vi "GDSIconEditor_HeaderEditorDialog.vi"(1 "BodyBackGround":u32(colorbox), 2 "HeaderText":string, 5 "error in (no error)":errorcluster, 6 "HeaderIconIn":u8[][](array[numeric]) format="%x", 7 "Type":T2, 8 "FrameThickness(1)":u32=1, 9 "ClassBodyIcon":string, 10 "FrameColor":u32(colorbox)) -> (15 "Cancelled":bool, 16 "FrameColorOut":u32(colorbox), 17 "FrameThicknessOut":u32=1, 18 "HeaderIconOut":u8[][](array[numeric]) format="%x", 19 "error out":errorcluster)   [LabVIEW 2020]
uses:
  <resource>/Framework/Providers/Open_GDS/ClassProviders/Common/LvIcon_class/GDSLvIcon_ColorControl.ctl
  <resource>/Framework/Providers/Open_GDS/ClassProviders/Common/LvIcon_class/GDSLvIcon_Type.ctl
  <vilib>/Utility/miscctls.llb/LVPoint32TypeDef.ctl
  <resource>/Framework/Providers/Open_GDS/ClassProviders/Common/LvIcon_class/GDSLvIcon_ClassColorTypes.ctl
  <resource>/Framework/Providers/Open_GDS/ClassProviders/Common/LvIcon_class/subvis/GDSLvIcon_TextDataType.ctl
  <resource>/Framework/Providers/Open_GDS/ClassProviders/Common/LvIcon_class/GDSLvIcon_WordCompressionType.ctl
  <resource>/Framework/Providers/Open_GDS/ClassProviders/Common/LvIcon_class/GDSLvIcon_TextAlignment.ctl
  <vilib>/event_ctls.llb/lveventtype.ctl
  <vilib>/Analysis/NI_AALBase.lvlib
panel:
  out "Coords 2":T1
  out "Coords":T1
  in  "_LastHeaders":picture[](array[picture]) caption="Last used headers"
  in  "Help":bool
  in  "Dice":cluster{"Boolean 2":bool, "Dice 2":bool}
  out "Icon Preview":picture
  in  "Frame":T3 caption="Color"
  in  "Thickness (pixels)":u8=3 min=1 max=3 step=1
  in  "Rows":enum16{"1 Row", "2 Rows", "3 Rows"}(ring)
  in  "Font Compression":enum16{"Auto", "On", "Off"}(ring)
  in  "CapitalOnly":bool=TRUE caption="Only use capital characters"
  in  "Height (pixels)":u8=9 min=5 max=19
  in  "Text":string="Endevo"
  in  "HeaderBk":T3 caption="Background"
  in  "HeaderText":T3 caption="Text"
  in  "OK":bool
  in  "Cancel":bool
  # "Header"
  # "Random color generation"
  # "Frame"
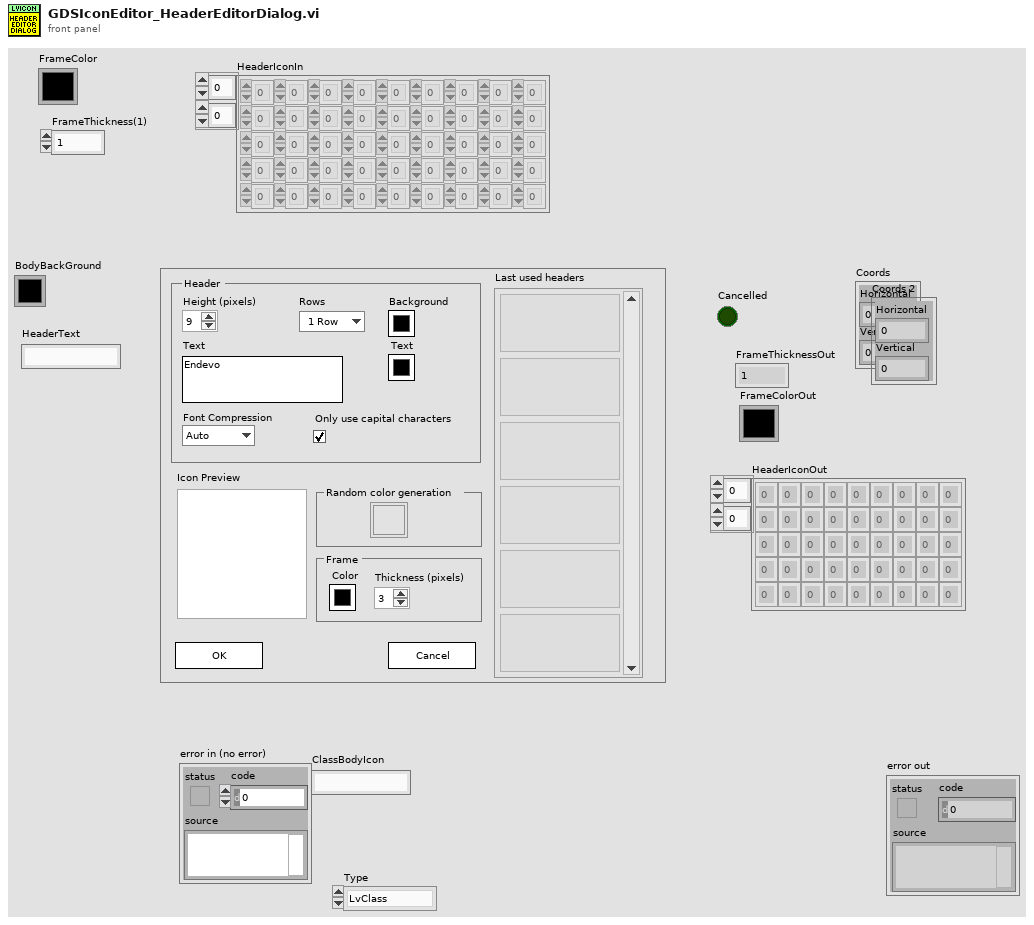
[diagram p1: front panel]
types:
  T1 = typedef "LVPoint32TypeDef.ctl" = cluster{"Horizontal":i32, "Vertical":i32}
  T2 = typedef "GDSLvIcon_Type.ctl" = enum16{"LvClass", "Library", "X-Control", "LvInterface"}
  T3 = typedef "GDSLvIcon_ColorControl.ctl" = cluster{"Decal":bool, "Color":u32}
  T4 = cluster{"Names":string[], "Headers":cluster{"Header":u8[][]}[]}
  T5 = typedef "GDSLvIcon_ClassColorTypes.ctl" = cluster{"Frame":u32, "Header Text Color":u32, "Header Background":u32, "BodyBackgroundPublic":u32, "BodyBackgroundProtected":u32, "BodyBackgroundPrivate":u32, "Body Text Color":u32, "Frame thickness":u8, "ProtectedPrivateSame":bool, "Icon Header Size":u8, "Font Compression":enum16{"Auto", "On", "Off"}, "CapitalOnly":bool}
  T6 = cluster{"Header":u8[][], "Cancel":bool, "Names":string[], "Headers":cluster{"Header":u8[][]}[]}
  T7 = cluster{"Selection Start":u32, "Selection End":u32}
  T8 = cluster{"left":i16, "top":i16, "right":i16, "bottom":i16}
  T9 = typedef "GDSLvIcon_TextDataType.ctl" = cluster{"Text":string, "Allow Only Capital Chars":bool, "Compression":T10, "Alignment":T11}
  T10 = typedef "GDSLvIcon_WordCompressionType.ctl" = enum16{"Auto", "On", "Off"}
  T11 = typedef "GDSLvIcon_TextAlignment.ctl" = enum16{"Center", "Left", "Right"}
  T12 = typedef "lveventtype.ctl" = enum32{"Null", "Timeout", "Annotation Menu Selection", "Annotation Menu Selection?", "App Instance Close", "App Instance Close?", "Autoscale Range Change", "Bookmark Info Change", "Cell Edit", "Cell Edit?", "Cursor Grab", "Cursor Grab?", "Cursor Menu Selection", "Cursor Menu Selection?", "Cursor Move", "Cursor Release", "Data Change", "Direction Change", "Display State Change", "Drag Ended", "Drag Enter", "Drag Leave", "Drag Over", "Drag Source Update", "Drag Starting", "Drag Starting?", "Drop", "Exec State Change", "Key Down", "Key Down?", "Key Repeat", "Key Repeat?", "Key Up", "Listbox Double Click", "Menu Activation?", "Menu Selection (App)", "Menu Selection? (App)", "Menu Selection (User)", "Mouse Down", "Mouse Down?", "Mouse Enter", "Mouse Leave", "Mouse Move", "Mouse Up", "Mouse Wheel", "NI Security User Change (App)", "Pane Size", "Panel Close", "Panel Close?", "Panel Resize", "Plot Attribute Change", "Scale Range Change", "Shortcut Menu Activation?", "Shortcut Menu Selection (App)", "Shortcut Menu Selection? (App)", "Shortcut Menu Selection (User)", "Tree Double Click", "Tree Drag", "Tree Drag?", "Tree Drop", "Tree Drop?", "Tree Item Close", "Tree Item Close?", "Tree Item Open", "Tree Item Open?", "User Event", "Value Change"}
  T13 = typedef "ColorControl.ctl" = cluster{"Decal":bool, "Color":u32}
  T14 = typedef "LVRectTypeDef.ctl" = cluster{"Left":i16, "Top":i16, "Right":i16, "Bottom":i16}
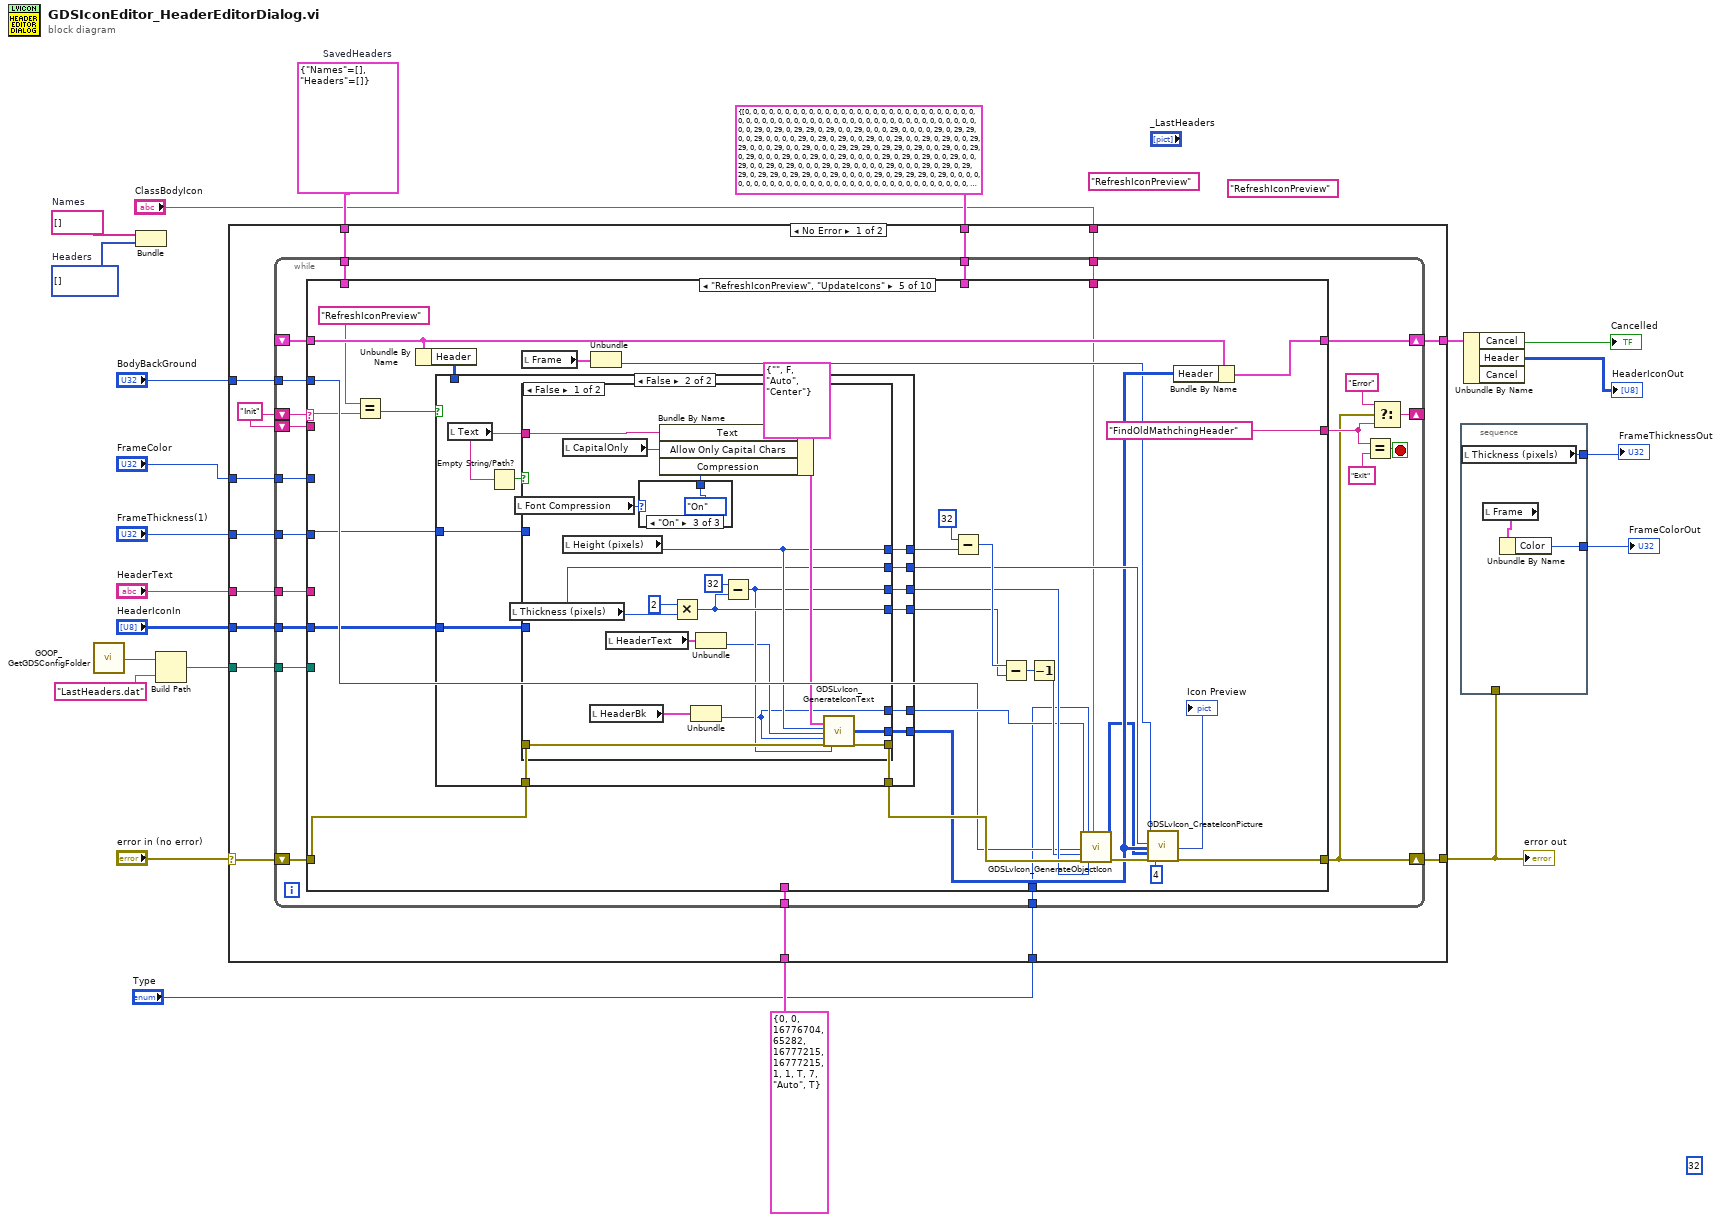
[diagram p0: block diagram]
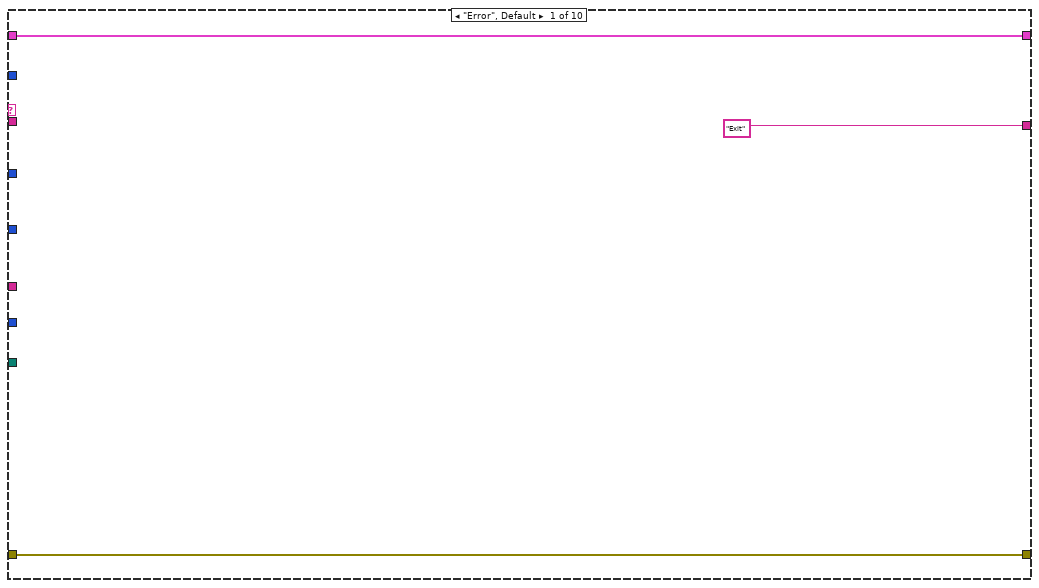
[diagram p2: hidden frame]
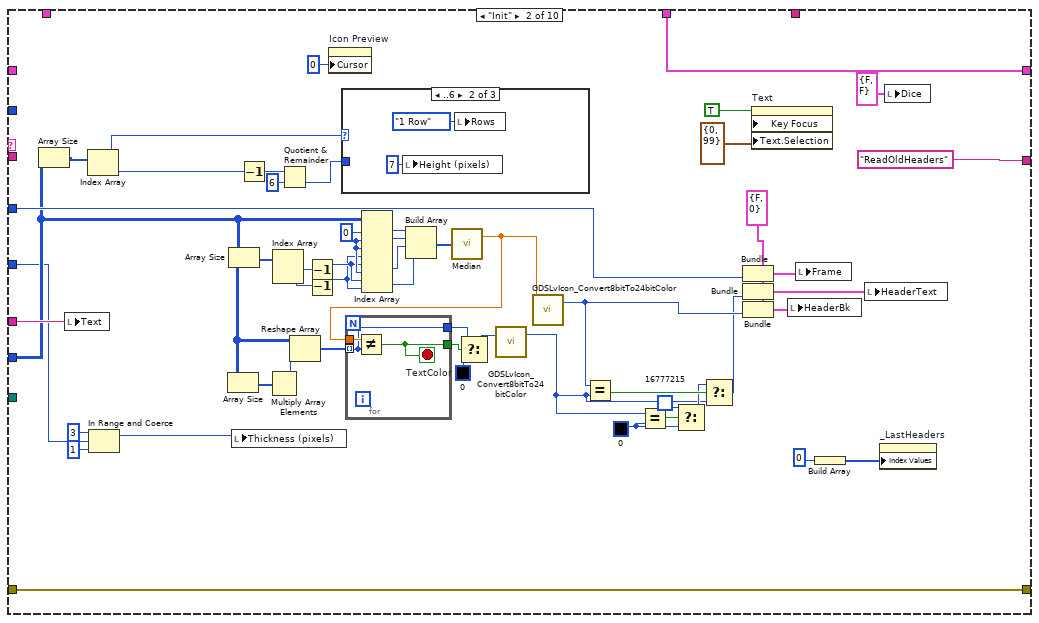
[diagram p3: hidden frame]
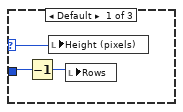
[diagram p4: hidden frame]
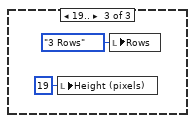
[diagram p5: hidden frame]
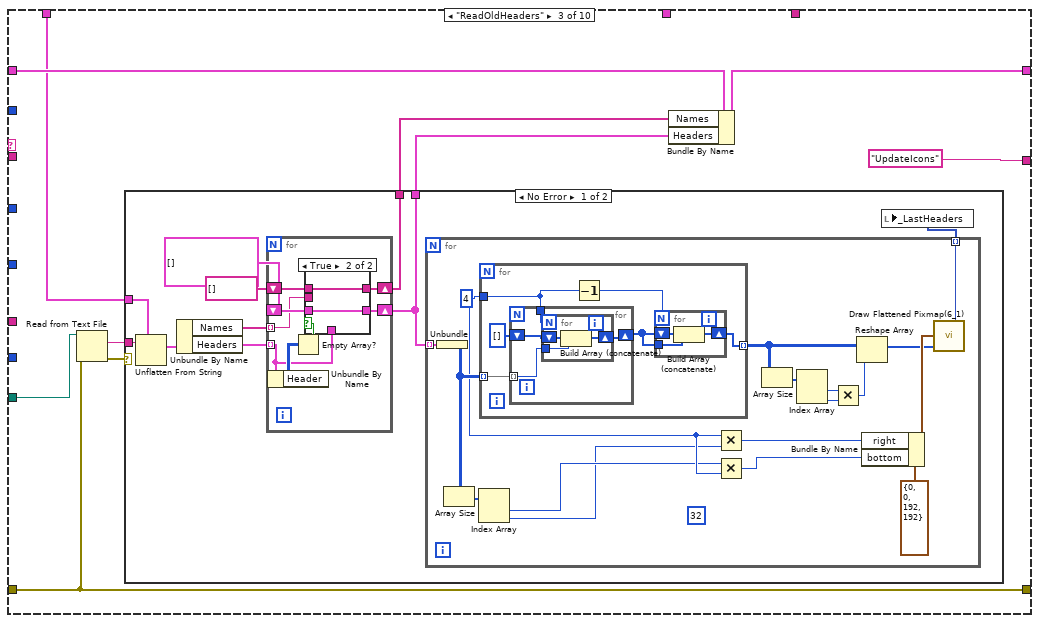
[diagram p6: hidden frame]
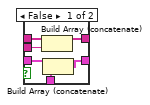
[diagram p7: hidden frame]
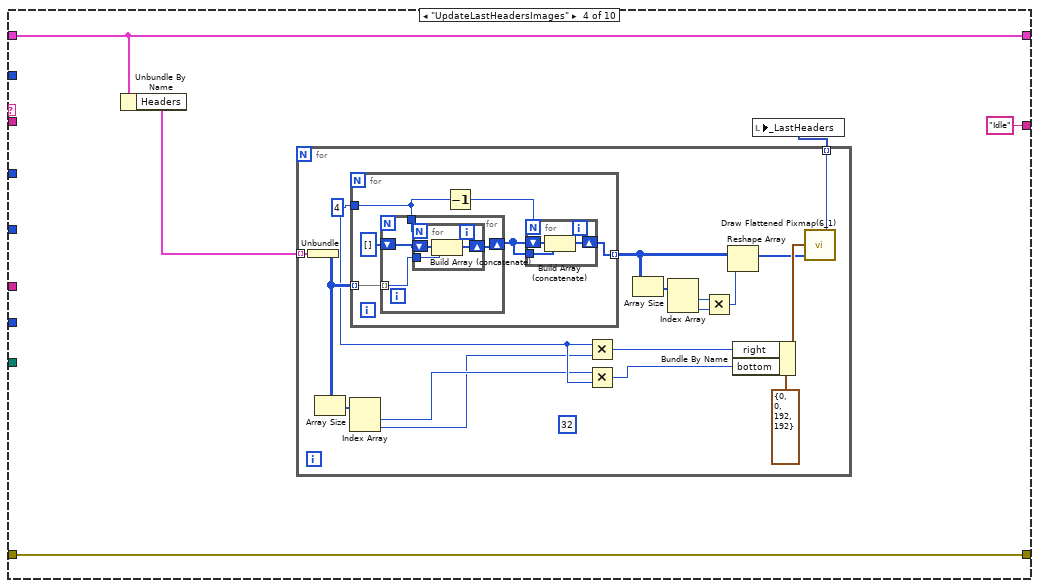
[diagram p9: hidden frame]
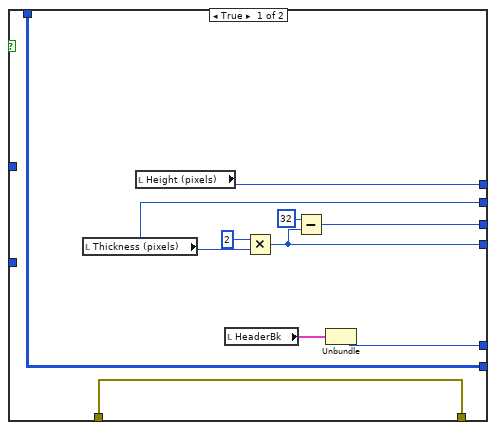
[diagram p10: hidden frame]
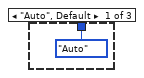
[diagram p11: hidden frame]
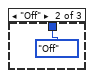
[diagram p12: hidden frame]
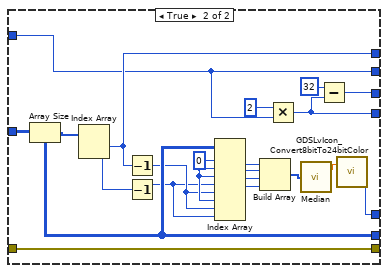
[diagram p13: hidden frame]
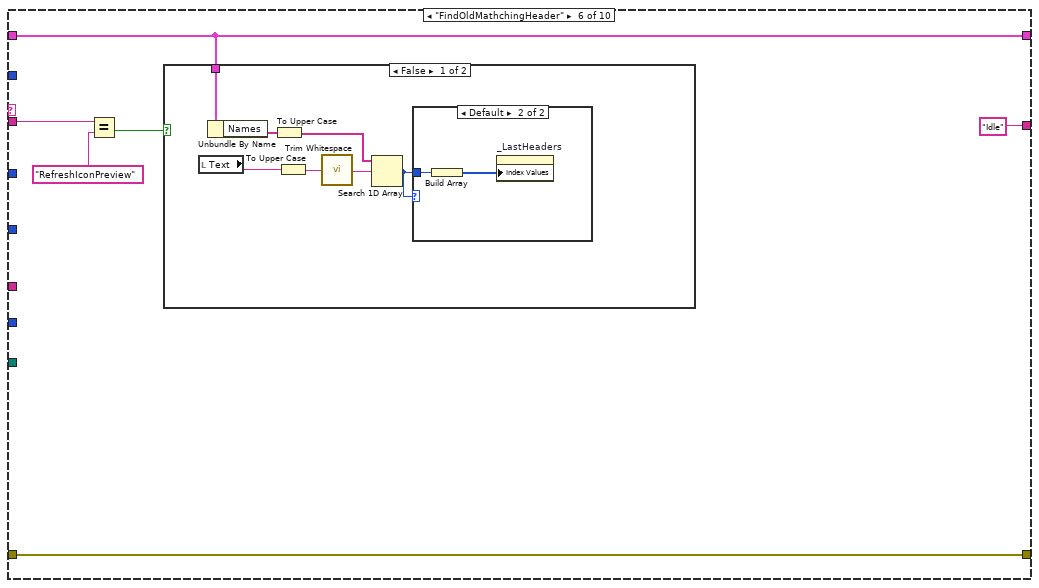
[diagram p14: hidden frame]
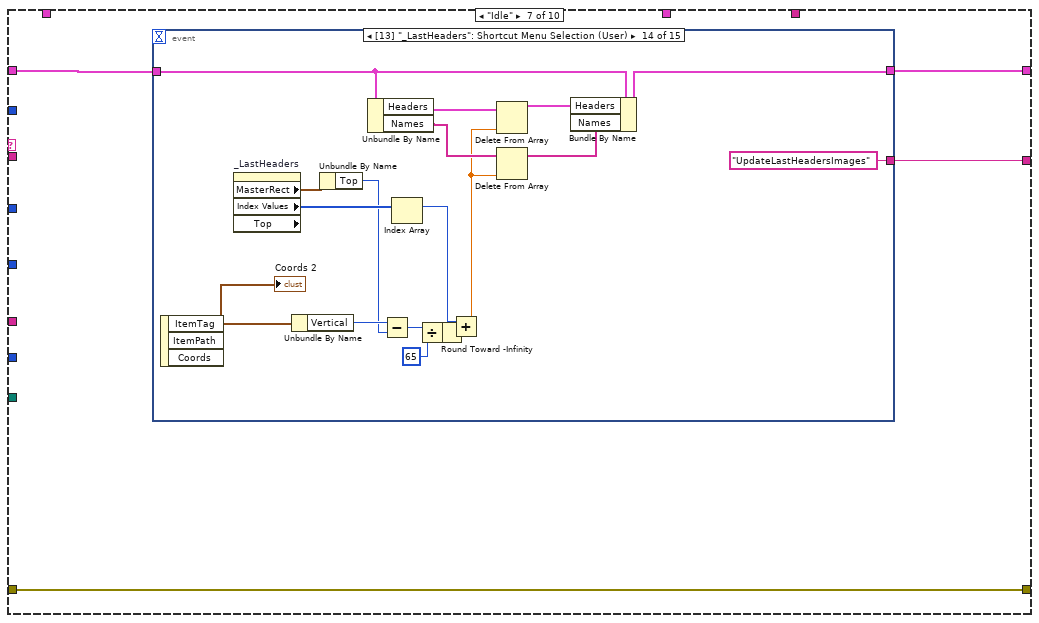
[diagram p17: hidden frame]
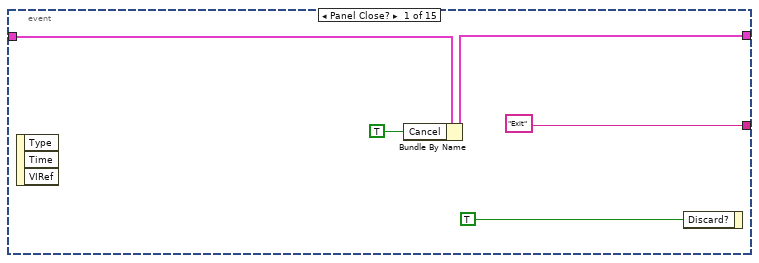
[diagram p18: hidden frame]
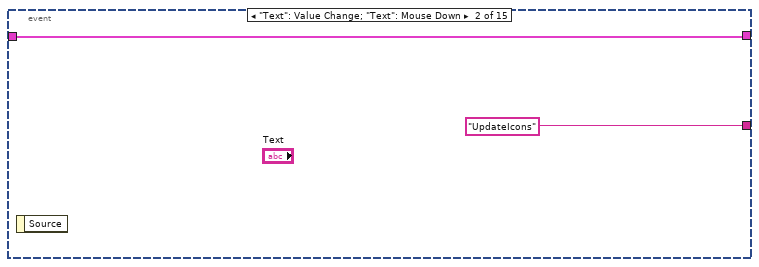
[diagram p19: hidden frame]
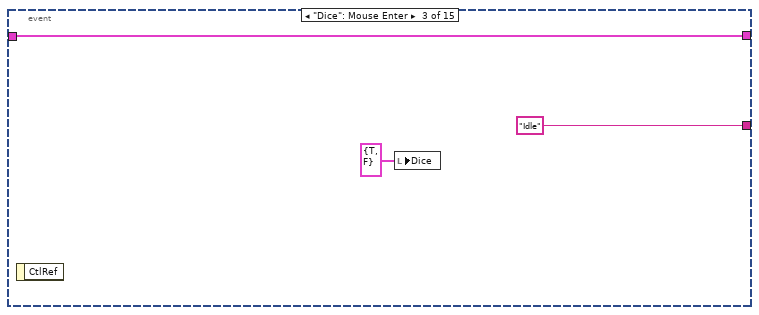
[diagram p20: hidden frame]
diagram:
  (unwired) "RefreshIconPreview"
  (unwired) "RefreshIconPreview"
  w2 = T4 {"Names"=[], "Headers"=[]}  # SavedHeaders
  (unwired) i16 32 ("bottom")
  w4 = picture[] []  # Headers
  w3 = string[] []  # Names
  n1 = call <resource>:"GOOP_GetGDSConfigFolder.vi"() -> ("GDSFolderPath"=w6:path)
  n2 = Bundle("Names"=w3, "Headers"=w4) -> ()  [unwired: 1 in, 1 out]
  n3 = Build Path(base path=w6, name or relative path="LastHeaders.dat") -> (appended path=w5:path)
  n4 = case shown="No Error" "error in (no error)" {
    selector: "error in (no error)" -> [w37 w575]
    tunnel: [w36 w575] -> w12
    tunnel: "BodyBackGround" -> [w35 _]
    tunnel: T6 {"Header"=[[0, 0, 0, 0, 0, 0, 0, 0, 0, 0, 0, 0, 0, 0, 0, 0, 0, 0, 0, 0, 0, 0, 0, 0, 0, 0, 0, 0, 0, 0], [0, 0, 0, 0, 0, 0, 0, 0, 0, 0, 0, 0, 0, 0, 0, 0, 0, 0, 0, 0, 0, 0, 0, 0, 0, 0, 0, 0, 0, 0], [0, 29, 0, 29, 0, 29, 29, 0, 29, 0, 0, 29, 0, 0, 0, 29, 0, 0, 0, 0, 29, 0, 29, 29, 0, 0, 29, 0, 0, 0], [0, 29, 0, 29, 0, 29, 0, 0, 29, 0, 0, 29, 0, 0, 29, 0, 29, 0, 0, 29, 29, 0, 0, 0, 29, 0, 0, 29, 0, 0], [0, 29, 29, 29, 0, 29, 29, 0, 29, 0, 0, 29, 0, 0, 29, 0, 29, 0, 0, 0, 29, 0, 0, 29, 0, 0, 29, 0, 0, 0], [0, 29, 0, 29, 0, 29, 0, 0, 29, 0, 0, 29, 0, 0, 29, 0, 29, 0, 0, 0, 29, 0, 29, 0, 0, 0, 0, 29, 0, 0], [0, 29, 0, 29, 0, 29, 29, 0, 29, 29, 0, 29, 29, 0, 0, 29, 0, 0, 0, 0, 29, 0, 29, 29, 29, 0, 29, 0, 0, 0], [0, 0, 0, 0, 0, 0, 0, 0, 0, 0, 0, 0, 0, 0, 0, 0, 0, 0, 0, 0, 0, 0, 0, 0, 0, 0, 0, 0, 0, 0], [0, 0, 0, 0, 0, 0, 0, 0, 0, 0, 0, 0, 0, 0, 0, 0, 0, 0, 0, 0, 0, 0, 0, 0, 0, 0, 0, 0, 0, 0]], "Cancel"=FALSE, "Names"=[], "Headers"=[]} -> [w34 _]
    tunnel: T5 {"Frame"=0, "Header Text Color"=0, "Header Background"=16776704, "BodyBackgroundPublic"=65282, "BodyBackgroundProtected"=16777215, "BodyBackgroundPrivate"=16777215, "Body Text Color"=1, "Frame thickness"=1, "ProtectedPrivateSame"=TRUE, "Icon Header Size"=7, "Font Compression"=enum."Auto", "CapitalOnly"=TRUE} ("type") -> [w33 _]
    tunnel: "FrameThickness(1)" -> [w32 _]
    tunnel: "FrameColor" -> [w31 _]
    tunnel: "HeaderText" -> [w30 _]
    tunnel: [w29 _] -> w15
    tunnel: "HeaderIconIn" -> [w28 _]
    tunnel: "Type" -> [w27 _]
    tunnel: w5 -> [w26 _]
    tunnel: w2 -> [w25 _]
    tunnel: "ClassBodyIcon" -> [w23 _]
    frame No Error {
      w24 = "Init"
      n5 = while {
        shift-right: [w52] -> w36
        shift-left: w37 -> [w59]
        shift-right: [w57] -> _
        shift-left: w24 -> [w58]
        shift-right: [w41] -> w29
        shift-left: _ -> [w51]
        tunnel: w35 -> [w50]
        tunnel: w34 -> [w49]
        tunnel: w33 -> [w48]
        tunnel: w32 -> [w47]
        tunnel: w31 -> [w46]
        tunnel: w30 -> [w45]
        tunnel: w28 -> [w44]
        tunnel: w27 -> [w43]
        tunnel: w26 -> [w42]
        tunnel: w25 -> [w40]
        shift-left: w24 -> [w39]
        tunnel: w23 -> [w38]
        stop <- w56 stop-if-true
        n6 = case shown="\"RefreshIconPreview\", \"UpdateIcons\"" w58 {
          selector: w58 -> [_ _ _ _ w236 _ _ _ _ _]
          tunnel: w59 -> [w62 w105 w127 w197 w262 w330 w344 w457 w515 w532]
          tunnel: [w62 w105 w127 w197 w254 w330 w344 w457 w515 w532] -> w52
          tunnel: ["Exit" "ReadOldHeaders" "UpdateIcons" "Idle" "FindOldMathchingHeader" "Idle" w345 "RefreshIconPreview" "UpdateIcons" "Exit"] -> w53
          tunnel: w51 -> [w60 _ w130 w195 w237 w331 w343 w489 w530 w540]
          tunnel: w50 -> [_ _ _ _ w241 _ _ _ _ _]
          tunnel: w49 -> [_ w104 _ _ _ _ _ _ _ _]
          tunnel: w48 -> [_ _ _ _ _ _ _ _ _ _]
          tunnel: w47 -> [_ w69 _ _ w239 _ _ _ _ _]
          tunnel: w46 -> [_ w108 _ _ _ _ _ _ _ _]
          tunnel: w45 -> [_ w103 _ _ _ _ _ _ _ _]
          tunnel: w44 -> [_ w75 _ _ w240 _ _ _ _ _]
          tunnel: w43 -> [_ _ _ _ w238 _ _ _ _ _]
          tunnel: w42 -> [_ _ w133 _ _ _ _ _ _ w534]
          tunnel: [w60 w104 w129 w195 w248 w331 w342 w489 w530 w540] -> w41
          tunnel: w40 -> [_ _ w125 _ _ _ _ _ _ w535]
          tunnel: w39 -> [_ _ _ _ _ w329 _ _ _ _]
          tunnel: w38 -> [_ _ _ _ w233 _ _ _ _ _]
          frame "Error", Default {
          }
          frame "Init" {
            w109 = T3 {"Decal"=FALSE, "Color"=0} ("Frame")
            w76 = u32 0  # TextColor
            w90 = 0 ("index (row)")
            w70 = u32 0
            n7 = Array Size(array=w75) -> (size(s)=w102:i32[])
            n8 = local write "Text"(w103) -> ()
            n9 = Index Array(array=w102) -> (element=w99:i32)  [unwired: 1 in]
            n10 = In Range and Coerce(upper limit=u32 3, x=w69, lower limit=u32 1) -> (coerced(x)=w66:u32)  [unwired: 1 out]
            n11 = Array Size(array=w75) -> (size(s)=w82:i32[])
            n12 = Array Size(array=w75) -> (size(s)=w93:i32[])
            n13 = local write "Thickness (pixels)"(w66) -> ()
            n14 = Decrement(x=w99) -> (x-1=w101:i32)
            n15 = Multiply Array Elements(1:w82) -> (0:w80:i32)
            n16 = Index Array(array=w93) -> (element #1=w92:i32, element #2=w91:i32)  [unwired: 2 in]
            n17 = Quotient & Remainder(x=w101, y=6) -> (floor(x/y)=w98:i32)  [unwired: 1 out]
            n18 = Reshape Array(w75, w80) -> (w81:u8[])
            n19 = Decrement(x=w92) -> (x-1=w89:i32)
            n20 = Decrement(x=w91) -> (x-1=w88:i32)
            n21 = property on="Icon Preview" class="Pict"("Cursor"=0) -> ()  [unwired: 2 in, 2 out]
            n22 = case shown="..6" w99 {
              selector: w99 -> [w120 _ _]
              tunnel: w98 -> [w119 _ _]
              frame Default {
                n23 = Decrement(x=w119) -> (x-1=w118:i32)
                n24 = local write "Height (pixels)"(w120) -> ()
                n25 = local write "Rows"(w118) -> ()
              }
              frame ..6 {
                n26 = local write "Height (pixels)"(u8 7 ("Height (pixels)")) -> ()
                n27 = local write "Rows"(enum16{"1 Row", "2 Rows", "3 Rows"}."1 Row" ("Rows")) -> ()
              }
              frame 19.. {
                n28 = local write "Height (pixels)"(u8 19 ("Height (pixels)")) -> ()
                n29 = local write "Rows"(enum16{"1 Row", "2 Rows", "3 Rows"}."3 Rows" ("Rows")) -> ()
              }
            }
            n30 = Index Array(array=w75, index (row) #1=w90, index (col) #1=w90, index (row) #2=w90, index (col) #2=w88, index (row) #3=w89, index (col) #3=w90, index (row) #4=w89, index (col) #4=w88) -> (element #1=w87:u8, element #2=w86:u8, element #3=w85:u8, element #4=w84:u8)
            n31 = Build Array(w87, w86, w85, w84) -> (w83:u8[])
            n32 = call <vilib>:"Median.vi"("X"=w83) -> ("median"=w74:dbl)  [unwired: 1 out]
            n33 = for {
              tunnel: w81 -> [w116] mode=indexing
              tunnel: w74 -> [w117]
              tunnel: [w115] -> w78
              tunnel: [w116] -> w77
              stop <- w115 stop-if-true
              n34 = Not Equal?(x=w117, y=w116) -> (x != y?=w115:bool)
            }
            n35 = Select(t=w77, s=w78, f=w76) -> (s? t:f=w79:u32)
            n36 = call <resource>:"GDSLvIcon_Convert8bitTo24bitColor.vi"("Color8bit"=w79) -> ("Color24bit"=w71:u32)  [unwired: 17 in, 1 out]
            n37 = call <resource>:"GDSLvIcon_Convert8bitTo24bitColor.vi"("Color8bit"=w74) -> ("Color24bit"=w73:u32)  [unwired: 17 in, 1 out]
            n38 = Equal?(x=w73, y=w71) -> (x = y?=w97:bool)
            n39 = Equal?(x=w71, y=w70) -> (x = y?=w96:bool)
            n40 = Select(t=u32 16777215, s=w96, f=w70) -> (s? t:f=w94:u32)
            n41 = Select(t=w94, s=w97, f=w71) -> (s? t:f=w72:u32)
            n42 = Bundle(cluster=w109, "Color"=w108) -> (w112:T3)  [unwired: 1 in]
            n43 = Bundle(cluster=w109, "Color"=w72) -> (w111:T3)  [unwired: 1 in]
            n44 = Bundle(cluster=w109, "Color"=w73) -> (w110:T3)  [unwired: 1 in]
            n45 = property on="Text" class="Str"("Key Focus"=TRUE, "Text.Selection"=T7 {"Selection Start"=0, "Selection End"=99}) -> ()  [unwired: 2 in, 2 out]
            n46 = local write "HeaderBk"(w110) -> ()
            n47 = local write "Frame"(w112) -> ()
            n48 = Build Array(u32 0) -> (w65:u32[])
            n49 = local write "HeaderText"(w111) -> ()
            n50 = property on="_LastHeaders" class="Arr (strict)"("Index Values"=w65) -> ()  [unwired: 2 in, 2 out]
            n51 = local write "Dice"(cluster{"Boolean 2":bool, "Dice":bool} {"Boolean 2"=FALSE, "Dice"=FALSE} ("Dice")) -> ()
          }
          frame "ReadOldHeaders" {
            n52 = Read from Text File(file (use dialog)=w133, error in=w127) -> (text=w131:string, error out=w132:errorcluster)  [unwired: 2 in, 2 out]
            n53 = case shown="No Error" w132 {
              tunnel: w131 -> [w144 _]
              tunnel: w125 -> [w143 _]
              tunnel: [w135 _] -> w128
              tunnel: [w136 _] -> w126
              frame No Error {
                n54 = Unflatten From String(type=w143, binary string=w144) -> (value=w142:T4)  [unwired: 3 in, 2 out]
                n55 = Unbundle By Name(w142) -> ("Names"=w140:string[], "Headers"=w139:cluster{"Header":u8[][]}[])
                n56 = for {
                  tunnel: w140 -> [w147] mode=indexing
                  tunnel: w139 -> [w145] mode=indexing
                  shift-right: [w148] -> w135
                  shift-left: string[] [] -> [w150]
                  shift-right: [w146] -> w136
                  shift-left: cluster{"Header":u8[][]}[] [] -> [w149]
                  n57 = Unbundle By Name(w145) -> ("Header"=w152:u8[][])
                  n58 = Empty Array?(array=w152) -> (empty?=w151:bool)
                  n59 = case shown="True" w151 {
                    tunnel: w150 -> [w157 w159]
                    tunnel: w149 -> [w155 w160]
                    tunnel: [w158 w159] -> w148
                    tunnel: w147 -> [w156 _]
                    tunnel: [w154 w160] -> w146
                    tunnel: w145 -> [w153 _]
                    frame False {
                      n60 = Build Array (concatenate)(w157, w156) -> (w158:string[])
                      n61 = Build Array (concatenate)(w155, w153) -> (w154:cluster{"Header":u8[][]}[])
                    }
                    frame True {
                    }
                  }
                }
                n62 = for {
                  tunnel: w136 -> [w177] mode=indexing
                  tunnel: [w167] -> w141 mode=indexing
                  w164 = 4 ("BigSizeIcon(x6)")
                  (unwired) 32 ("y")
                  n63 = Unbundle(w177) -> ("Header"=w165:u8[][])
                  n64 = Array Size(array=w165) -> (size(s)=w166:i32[])
                  n65 = Index Array(array=w166) -> (element #1=w162:i32, element #2=w161:i32)  [unwired: 2 in]
                  n66 = for {
                    tunnel: w165 -> [w183] mode=indexing
                    tunnel: [w181] -> w172 mode=indexing
                    tunnel: w164 -> [w178]
                    n67 = for {
                      tunnel: w183 -> [w190] mode=indexing
                      shift-right: [w188] -> w180
                      shift-left: u8[] [] -> [w189]
                      tunnel: w178 -> [w187]
                      n68 = for {
                        N: w187 -> [_]
                        tunnel: w190 -> [w193]
                        shift-right: [w191] -> w188
                        shift-left: w189 -> [w192]
                        n69 = Build Array (concatenate)(w192, w193) -> (w191:u8[])
                      }
                    }
                    n70 = Decrement(x=w178) -> (x-1=w179:i32)
                    n71 = for {
                      N: w179 -> [_]
                      tunnel: w180 -> [w186]
                      shift-right: [w184] -> w181
                      shift-left: w180 -> [w185]
                      n72 = Build Array (concatenate)(w185, w186) -> (w184:u8[])
                    }
                  }
                  n73 = Multiply(x=w164, y=w161) -> (x*y=w176:i32)
                  n74 = Multiply(x=w162, y=w164) -> (x*y=w163:i32)
                  n75 = Array Size(array=w172) -> (size(s)=w168:i32[])
                  n76 = Index Array(array=w168) -> (element #1=w170:i32, element #2=w169:i32)  [unwired: 2 in]
                  n77 = Multiply(x=w170, y=w169) -> (x*y=w171:i32)
                  n78 = Reshape Array(w172, w171) -> (w173:u8[])
                  n79 = Bundle By Name(cluster=T8 {"left"=0, "top"=0, "right"=192, "bottom"=192} ("rect"), "right"=w176, "bottom"=w163) -> (w175:T8)
                  n80 = call <vilib>:"Draw Flattened Pixmap(6_1).vi"("rect"=w175, "flattened pixmap data"=w173) -> ("new picture"=w167:picture)  [unwired: 7 in]
                }
                n81 = local write "_LastHeaders"(w141) -> ()
              }
              frame Error {
              }
            }
            n82 = Bundle By Name(cluster=w130, "Names"=w128, "Headers"=w126) -> (w129:T6)
          }
          frame "UpdateLastHeadersImages" {
            n83 = Unbundle By Name(w195) -> ("Headers"=w196:cluster{"Header":u8[][]}[])
            n84 = for {
              tunnel: w196 -> [w215] mode=indexing
              tunnel: [w205] -> w198 mode=indexing
              w202 = 4 ("BigSizeIcon(x6)")
              (unwired) 32 ("y")
              n85 = Unbundle(w215) -> ("Header"=w203:u8[][])
              n86 = Array Size(array=w203) -> (size(s)=w204:i32[])
              n87 = Index Array(array=w204) -> (element #1=w200:i32, element #2=w199:i32)  [unwired: 2 in]
              n88 = for {
                tunnel: w203 -> [w221] mode=indexing
                tunnel: [w219] -> w210 mode=indexing
                tunnel: w202 -> [w216]
                n89 = for {
                  tunnel: w221 -> [w228] mode=indexing
                  shift-right: [w226] -> w218
                  shift-left: u8[] [] -> [w227]
                  tunnel: w216 -> [w225]
                  n90 = for {
                    N: w225 -> [_]
                    tunnel: w228 -> [w231]
                    shift-right: [w229] -> w226
                    shift-left: w227 -> [w230]
                    n91 = Build Array (concatenate)(w230, w231) -> (w229:u8[])
                  }
                }
                n92 = Decrement(x=w216) -> (x-1=w217:i32)
                n93 = for {
                  N: w217 -> [_]
                  tunnel: w218 -> [w224]
                  shift-right: [w222] -> w219
                  shift-left: w218 -> [w223]
                  n94 = Build Array (concatenate)(w223, w224) -> (w222:u8[])
                }
              }
              n95 = Multiply(x=w202, y=w199) -> (x*y=w214:i32)
              n96 = Multiply(x=w200, y=w202) -> (x*y=w201:i32)
              n97 = Array Size(array=w210) -> (size(s)=w206:i32[])
              n98 = Index Array(array=w206) -> (element #1=w208:i32, element #2=w207:i32)  [unwired: 2 in]
              n99 = Multiply(x=w208, y=w207) -> (x*y=w209:i32)
              n100 = Reshape Array(w210, w209) -> (w211:u8[])
              n101 = Bundle By Name(cluster=T8 {"left"=0, "top"=0, "right"=192, "bottom"=192} ("rect"), "right"=w214, "bottom"=w201) -> (w213:T8)
              n102 = call <vilib>:"Draw Flattened Pixmap(6_1).vi"("rect"=w213, "flattened pixmap data"=w211) -> ("new picture"=w205:picture)  [unwired: 7 in]
            }
            n103 = local write "_LastHeaders"(w198) -> ()
          }
          frame "RefreshIconPreview", "UpdateIcons" {
            n104 = Equal?(x="RefreshIconPreview", y=w236) -> (x = y?=w232:bool)
            n105 = Unbundle By Name(w237) -> ("Header"=w234:u8[][])
            n106 = case shown="False" w232 {
              tunnel: w262 -> [w266 w284]
              tunnel: [w266 w283] -> w260
              tunnel: [w272 w282] -> w256
              tunnel: [w271 w281] -> w252
              tunnel: [w270 w280] -> w251
              tunnel: [w269 w279] -> w250
              tunnel: [w265 w278] -> w247
              tunnel: [w263 w277] -> w243
              tunnel: w240 -> [_ w274]
              tunnel: w239 -> [_ w273]
              tunnel: w234 -> [w265 _]
              frame True {
                n107 = local read "Thickness (pixels)"() -> (w270:u8)
                n108 = local read "Height (pixels)"() -> (w272:u8)
                n109 = local read "HeaderBk"() -> (w264:T3)
                n110 = Multiply(x=u8 2, y=w270) -> (x*y=w271:u8)
                n111 = Subtract(x=32, y=w271) -> (x-y=w269:i32)
                n112 = Unbundle(w264) -> ("Color"=w263:u32)  [unwired: 1 out]
              }
              frame False {
                n113 = local read "Text"() -> (w275:string)
                n114 = Empty String/Path?(string/path=w275) -> (empty?=w276:bool)
                n115 = case shown="False" w276 {
                  tunnel: w284 -> [w303 w326]
                  tunnel: [w298 w326] -> w283
                  tunnel: [w296 w320] -> w282
                  tunnel: [w294 w321] -> w281
                  tunnel: [w292 w309] -> w280
                  tunnel: [w291 w322] -> w279
                  tunnel: [w290 w318] -> w278
                  tunnel: [w286 w307] -> w277
                  tunnel: w275 -> [w285 _]
                  tunnel: w274 -> [_ w318]
                  tunnel: w273 -> [_ w309]
                  frame False {
                    n116 = local read "Thickness (pixels)"() -> (w292:u8)
                    n117 = local read "Font Compression"() -> (w301:enum16{"Auto", "On", "Off"})
                    n118 = local read "CapitalOnly"() -> (w293:bool)
                    n119 = local read "Height (pixels)"() -> (w296:u8)
                    n120 = local read "HeaderBk"() -> (w287:T3)
                    n121 = local read "HeaderText"() -> (w289:T3)
                    n122 = case shown="\"On\"" w301 {
                      tunnel: [enum16{"Auto", "On", "Off"}."Auto" ("Compression") enum16{"Auto", "On", "Off"}."Off" ("Compression") enum16{"Auto", "On", "Off"}."On" ("Compression")] -> w302
                      frame "Auto", Default {
                      }
                      frame "Off" {
                      }
                      frame "On" {
                      }
                    }
                    n123 = Bundle By Name(cluster=T9 {"Text"="", "Allow Only Capital Chars"=FALSE, "Compression"=enum."Auto", "Alignment"=enum."Center"} ("Text"), "Text"=w285, "Allow Only Capital Chars"=w293, "Compression"=w302) -> (w299:T9)
                    n124 = Multiply(x=u8 2, y=w292) -> (x*y=w294:u8)
                    n125 = Unbundle(w287) -> ("Color"=w286:u32)  [unwired: 1 out]
                    n126 = Unbundle(w289) -> ("Color"=w288:u32)  [unwired: 1 out]
                    n127 = Subtract(x=32, y=w294) -> (x-y=w291:i32)
                    n128 = call <resource>:"GDSLvIcon_GenerateIconText.vi"("Text"=w299, "TextPixelHeight(5-30)"=w296, "Foreground color"=w288, "Background color"=w286, "error in (no error)"=w303, "Text Pixel width(32-FrameThicknes*2))"=w291) -> ("TextOut"=w290:u8[][], "error out"=w298:errorcluster)  [unwired: 9 in, 3 out]
                  }
                  frame True {
                    w317 = 0 ("index (row)")
                    n129 = Array Size(array=w318) -> (size(s)=w325:i32[])
                    n130 = Index Array(array=w325) -> (element #1=w320:i32, element #2=w319:i32)  [unwired: 2 in]
                    n131 = Decrement(x=w320) -> (x-1=w316:i32)
                    n132 = Decrement(x=w319) -> (x-1=w315:i32)
                    n133 = Index Array(array=w318, index (row) #1=w317, index (col) #1=w317, index (row) #2=w317, index (col) #2=w315, index (row) #3=w316, index (col) #3=w317, index (row) #4=w316, index (col) #4=w315) -> (element #1=w314:u8, element #2=w313:u8, element #3=w312:u8, element #4=w311:u8)
                    n134 = Build Array(w314, w313, w312, w311) -> (w310:u8[])
                    n135 = Multiply(x=u8 2, y=w309) -> (x*y=w321:u32)
                    n136 = call <vilib>:"Median.vi"("X"=w310) -> ("median"=w308:dbl)  [unwired: 1 out]
                    n137 = Subtract(x=32, y=w321) -> (x-y=w322:u32)
                    n138 = call <resource>:"GDSLvIcon_Convert8bitTo24bitColor.vi"("Color8bit"=w308) -> ("Color24bit"=w307:u32)  [unwired: 17 in, 1 out]
                  }
                }
              }
            }
            n139 = local read "Frame"() -> (w244:T3)
            n140 = Unbundle(w244) -> ("Color"=w245:u32)  [unwired: 1 out]
            n141 = Subtract(x=32, y=w256) -> (x-y=w259:i32)
            n142 = Subtract(x=w259, y=w252) -> (x-y=w258:u32)
            n143 = Decrement(x=w258) -> (x-1=w249:u32)
            n144 = call <resource>:"GDSLvIcon_GenerateObjectIcon.vi"("HeaderColor"=w243, "BackgroundColor"=w241, "Height"=w249, "error in (no error)"=w260, "Type"=w238, "Width(30)"=w250, "ClassBodyIcon"=w233) -> ("BodyIconOut"=w246:u8[][], "error out"=w255:errorcluster)  [unwired: 11 in]
            n145 = call <resource>:"GDSLvIcon_CreateIconPicture.vi"("FrameColor"=w245, "FrameThickness(1)"=w251, "HeaderIconIn"=w247, "BodyIconIn"=w246, "error in (no error)"=w255, "BigSizeIcon(x6)"=4) -> ("LargeIconPictureOut(x6)"=→"Icon Preview":picture, "error out"=w254:errorcluster)  [unwired: 8 in, 4 out]
            n146 = Bundle By Name(cluster=w237, "Header"=w247) -> (w248:T6)
          }
          frame "FindOldMathchingHeader" {
            n147 = Equal?(x=w329, y="RefreshIconPreview") -> (x = y?=w327:bool)
            n148 = case shown="False" w327 {
              tunnel: w331 -> [w339 _]
              frame False {
                n149 = local read "Text"() -> (w337:string)
                n150 = Unbundle By Name(w339) -> ("Names"=w338:string[])
                n151 = To Upper Case(1:w338) -> (0:w334:string[])
                n152 = To Upper Case(1:w337) -> (0:w336:string)
                n153 = call <vilib>:"Trim Whitespace.vi"("string"=w336) -> ("trimmed string"=w335:string)  [unwired: 1 in]
                n154 = Search 1D Array(1D array=w334, element=w335) -> (index of element=w333:i32)  [unwired: 1 in]
                n155 = case shown="Default" w333 {
                  tunnel: w333 -> [_ w341]
                  frame -1 {
                  }
                  frame Default {
                    n156 = Build Array(w341) -> (w340:i32[])
                    n157 = property on="_LastHeaders" class="Arr (strict)"("Index Values"=w340) -> ()  [unwired: 2 in, 2 out]
                  }
                }
              }
              frame True {
              }
            }
          }
          frame "Idle" {
            n158 = event shown="[13] \"_LastHeaders\": Shortcut Menu Selection (User)" {
              selector: _ -> [_ _ _ _ _ _ _ _ _ _ _ _ _ _ _]
              dyn-events: _ -> [_ _ _ _ _ _ _ _ _ _ _ _ _ _ _]
              timeout: _ -> [_ _ _ _ _ _ _ _ _ _ _ _ _ _ _]
              tunnel: ["Exit" "UpdateIcons" "Idle" "Idle" "Idle" "RandomColors" "UpdateIcons" "Idle" "UpdateIcons" "RefreshIconPreview" "RefreshIconPreview" "UpdateLastHeaders" w398 "UpdateLastHeadersImages" "Exit"] -> w345
              tunnel: w343 -> [w348 w351 w355 w357 w360 w362 w364 w367 w375 w383 w385 w393 w396 w436 w451]
              tunnel: [w346 w351 w355 w357 w360 w362 w364 w367 w375 w383 w385 w393 w397 w435 w450] -> w342
              event Panel Close? {
                n159 = event-data() -> ()  [unwired: 1 in, 3 out]
                n160 = Bundle By Name(cluster=w348, "Cancel"=TRUE) -> (w346:T6)
                n161 = event-data("Discard?"=TRUE) -> ()  [unwired: 1 in, 1 out]
              }
              event "Text": Value Change; "Text": Mouse Down {
                n162 = event-data() -> ()  [unwired: 1 in, 1 out]
              }
              event "Dice": Mouse Enter {
                n163 = event-data() -> ()  [unwired: 1 in, 1 out]
                n164 = local write "Dice"(cluster{"Boolean 2":bool, "Dice":bool} {"Boolean 2"=TRUE, "Dice"=FALSE} ("Dice")) -> ()
              }
              event "Help": Value Change {
                n165 = event-data() -> ()  [unwired: 1 in, 6 out]
              }
              event "Dice": Mouse Leave {
                n166 = event-data() -> ()  [unwired: 1 in, 1 out]
                n167 = local write "Dice"(cluster{"Boolean 2":bool, "Dice":bool} {"Boolean 2"=FALSE, "Dice"=FALSE} ("Dice")) -> ()
              }
              event "Dice": Value Change {
                n168 = event-data() -> ()  [unwired: 1 in, 6 out]
                n169 = local write "Dice"(cluster{"Boolean 2":bool, "Dice":bool} {"Boolean 2"=TRUE, "Dice"=FALSE} ("Dice")) -> ()
              }
              event "CapitalOnly", "Font Compression": Value Change {
                n170 = event-data() -> ()  [unwired: 1 in, 1 out]
              }
              event Mouse Enter; Mouse Leave {
                n171 = event-data() -> ("Type"=w370:T12, "CtlRef"=w374:refnum<vi>)  [unwired: 1 in]
                n172 = Equal?(x=w370, y=lveventtype."Mouse Enter") -> (x = y?=w368:bool)
                n173 = property class="Clust (strict)"(reference=w374) -> (reference out=w373:refnum<vi>, "Value"=w372:T13)  [unwired: 1 in, 1 out]
                n174 = Bundle By Name(cluster=w372, "Decal"=w368) -> (w371:T13)
                n175 = property class="Clust (strict)"(reference=w373, "Value"=w371) -> ()  [unwired: 1 in, 2 out]
              }
              event "Rows": Value Change {
                n176 = event-data() -> ()  [unwired: 1 in, 1 out]
                n177 = case shown="\"1 Row\", Default" "Rows" {
                  tunnel: [u8 7 ("Icon Header Size") u8 13 ("Icon Header Size") u8 19 ("Icon Header Size")] -> w377
                  frame "1 Row", Default {
                  }
                  frame "2 Rows" {
                  }
                  frame "3 Rows" {
                  }
                }
                n178 = local write "Height (pixels)"(w377) -> ()
              }
              event "Thickness (pixels)": Value Change {
                (unwired) "UpdateIcons"
                n179 = event-data() -> ()  [unwired: 1 in, 1 out]
              }
              event "Height (pixels)": Value Change {
                (unwired) "UpdateIcons"
                n180 = event-data() -> ()  [unwired: 1 in, 1 out]
                n181 = Quotient & Remainder(x="Height (pixels)", y=u8 5) -> (floor(x/y)=w386:u8)  [unwired: 1 out]
                n182 = case shown="3.." w386 {
                  tunnel: [enum16{"1 Row", "2 Rows", "3 Rows"}."1 Row" ("Rows") enum16{"1 Row", "2 Rows", "3 Rows"}."2 Rows" ("Rows") enum16{"1 Row", "2 Rows", "3 Rows"}."3 Rows" ("Rows")] -> w387
                  frame 1, Default {
                  }
                  frame 2 {
                  }
                  frame 3.. {
                  }
                }
                n183 = local write "Rows"(w387) -> ()
              }
              event "OK": Value Change {
                n184 = event-data() -> ()  [unwired: 1 in, 6 out]
              }
              event "_LastHeaders": Mouse Down {
                n185 = event-data() -> ("Button"=w395:u16, "Coords"=w399:T1)  [unwired: 1 in]
                n186 = case shown="1" w395 {
                  tunnel: w399 -> [_ w419]
                  tunnel: ["Idle" w418] -> w398
                  tunnel: [w401 w417] -> w397
                  tunnel: w396 -> [w401 w411]
                  frame 0, Default {
                  }
                  frame 1 {
                    n187 = property on="_LastHeaders" class="Arr (strict)" props=["MasterRect", "Index Values", "Top"]() -> ("MasterRect"=w404:T14, "Index Values"=w412:u32[])  [unwired: 2 in, 3 out]
                    n188 = Unbundle By Name(w419) -> ("Vertical"=w416:i32)
                    n189 = Unbundle By Name(w411) -> ("Headers"=w410:cluster{"Header":u8[][]}[])
                    n190 = Unbundle By Name(w404) -> ("Top"=w403:i16)
                    n191 = Subtract(x=w416, y=w403) -> (x-y=w415:i32)
                    n192 = Index Array(array=w412) -> (element=w408:u32)  [unwired: 1 in]
                    n193 = Divide(x=w415, y=65) -> (x/y=w413:dbl)
                    n194 = Round Toward -Infinity(1:w413) -> (0:w402:dbl)
                    n195 = Add(x=w408, y=w402) -> (x+y=w409:dbl)
                    n196 = Index Array(array=w410, index=w409) -> (element=w407:cluster{"Header":u8[][]})
                    n197 = Unbundle By Name(w407) -> ("Header"=w406:u8[][])
                    n198 = Empty Array?(array=w406) -> (empty?=w405:bool)
                    n199 = case shown="False" w405 {
                      tunnel: ["HeaderOCR" "Idle"] -> w418
                      tunnel: [w425 w431] -> w417
                      tunnel: w411 -> [w424 w431]
                      tunnel: w406 -> [w423 _]
                      frame False {
                        n200 = Array Size(array=w423) -> (size(s)=w422:i32[])
                        n201 = Bundle By Name(cluster=w424, "Header"=w423) -> (w425:T6)
                        n202 = Index Array(array=w422) -> (element=w421:i32)  [unwired: 1 in]
                        n203 = case shown="17.., Default" w421 {
                          tunnel: [enum16{"1 Row", "2 Rows", "3 Rows"}."1 Row" ("Rows") enum16{"1 Row", "2 Rows", "3 Rows"}."2 Rows" ("Rows") enum16{"1 Row", "2 Rows", "3 Rows"}."3 Rows" ("Rows")] -> w420
                          frame ..10 {
                          }
                          frame 11..16 {
                          }
                          frame 17.., Default {
                          }
                        }
                        n204 = local write "Rows"(w420) -> ()
                        n205 = local write "Height (pixels)"(w421) -> ()
                      }
                      frame True {
                      }
                    }
                    "Coords" <- w419
                  }
                }
              }
              event "_LastHeaders": Shortcut Menu Selection (User) {
                n206 = event-data() -> ("Coords"=w438:T1)  [unwired: 1 in, 2 out]
                "Coords 2" <- w438
                n207 = property on="_LastHeaders" class="Arr (strict)" props=["MasterRect", "Index Values", "Top"]() -> ("MasterRect"=w441:T14, "Index Values"=w444:u32[])  [unwired: 2 in, 3 out]
                n208 = Unbundle By Name(w438) -> ("Vertical"=w448:i32)
                n209 = Unbundle By Name(w441) -> ("Top"=w440:i16)
                n210 = Unbundle By Name(w436) -> ("Headers"=w443:cluster{"Header":u8[][]}[], "Names"=w437:string[])
                n211 = Subtract(x=w448, y=w440) -> (x-y=w447:i32)
                n212 = Index Array(array=w444) -> (element=w442:u32)  [unwired: 1 in]
                n213 = Divide(x=w447, y=65) -> (x/y=w445:dbl)
                n214 = Round Toward -Infinity(1:w445) -> (0:w439:dbl)
                n215 = Add(x=w442, y=w439) -> (x+y=w432:dbl)
                n216 = Delete From Array(array=w443, index=w432) -> (array with subset deleted=w433:cluster{"Header":u8[][]}[])  [unwired: 1 in, 1 out]
                n217 = Delete From Array(array=w437, index=w432) -> (array with subset deleted=w434:string[])  [unwired: 1 in, 1 out]
                n218 = Bundle By Name(cluster=w436, "Headers"=w433, "Names"=w434) -> (w435:T6)
              }
              event "Cancel": Value Change {
                n219 = event-data() -> ()  [unwired: 1 in, 6 out]
                n220 = Bundle By Name(cluster=w451, "Cancel"=TRUE) -> (w450:T6)
              }
            }
          }
          frame "HeaderOCR" {
            w477 = 0 ("index (row)")
            w482 = u8 255  # Black(8bit)
            n221 = Unbundle By Name(w489) -> ("Header"=w455:u8[][])
            n222 = Array Size(array=w455) -> (size(s)=w480:i32[])
            n223 = Index Array(array=w480) -> (element #1=w479:i32, element #2=w478:i32)  [unwired: 2 in]
            n224 = Array Size(array=w455) -> (size(s)=w488:i32[])
            n225 = Decrement(x=w479) -> (x-1=w476:i32)
            n226 = Decrement(x=w478) -> (x-1=w475:i32)
            n227 = Multiply Array Elements(1:w488) -> (0:w486:i32)
            n228 = Index Array(array=w455) -> (element=w470:u8[])  [unwired: 2 in]
            n229 = Reshape Array(w455, w486) -> (w487:u8[])
            n230 = Index Array(array=w455, index (row) #1=0 ("index (row)"), index (col) #1=4 ("disabled index (col)"), index (row) #2=w477, index (col) #2=w477, index (row) #3=w477, index (col) #3=w475, index (row) #4=w476, index (col) #4=w477, index (row) #5=w476, index (col) #5=w475) -> (element #1=w463:u8, element #2=w474:u8, element #3=w473:u8, element #4=w472:u8, element #5=w471:u8)
            n231 = Decrement(x=w486) -> (x-1=w485:i32)
            n232 = Array Max & Min(array=w470) -> (max value=w467:u8, min value=w469:u8)  [unwired: 2 out]
            n233 = Equal?(x=w467, y=w469) -> (x = y?=w468:bool)
            n234 = Build Array(w463, w474, w473, w472, w471) -> (w462:u8[])
            n235 = for {
              tunnel: w462 -> [w494] mode=indexing
              shift-right: [w492] -> w460
              shift-left: u8[] [] -> [w493]
              n236 = case shown="255" w494 {
                selector: w494 -> [w495 _]
                tunnel: w493 -> [w497 w498]
                tunnel: [w496 w498] -> w492
                frame Default {
                  n237 = Build Array (concatenate)(w497, w495) -> (w496:u8[])
                }
                frame 255 {
                }
              }
            }
            n238 = call <vilib>:"Median.vi"("X"=w460) -> ("median"=w466:dbl)  [unwired: 1 out]
            n239 = To Unsigned Byte Integer(number=w466) -> (unsigned 8bit integer=w459:u8)
            n240 = Select(t=w467, s=w468, f=w459) -> (s? t:f=w454:u8)
            n241 = for {
              tunnel: w487 -> [w500] mode=indexing
              tunnel: w454 -> [w501]
              tunnel: w485 -> [_]
              tunnel: [w499] -> w484
              tunnel: [w500] -> w483
              stop <- w499 stop-if-true
              n242 = Not Equal?(x=w501, y=w500) -> (x != y?=w499:bool)
            }
            n243 = Select(t=w483, s=w484, f=w482) -> (s? t:f=w481:u8)
            n244 = Build Array(w481, w454) -> (w491:u8[])
            n245 = for {
              tunnel: [w504] -> w456
              tunnel: w455 -> [w506]
              tunnel: bool[] [FALSE, TRUE] -> [w505] mode=indexing
              tunnel: w491 -> [w502] mode=indexing
              stop <- w503 continue-if-true
              n246 = call <resource>:"GOOP_IconOCR.vi"("BackColor(T), TextColor(F)"=w505, "BackColor Or TextColor(8bit)"=w502, "Icon"=w506) -> ("String"=w504:string)  [unwired: 8 in]
              n247 = Empty String/Path?(string/path=w504) -> (empty?=w503:bool)
            }
            n248 = local write "Text"(w456) -> ()
          }
          frame "RandomColors" {
            w513 = T3 {"Decal"=FALSE, "Color"=0} ("Public")
            w516 = u32[] [15007601, 14876576, 16751729, 15400704, 15507711, 16775072, 12713864, 12124142, 16776704, 16754080, 16752888, 16383904, 7667498, 16754986, 12112639, 3079936, 16776704, 16745561, 9341183, 16746660, 16773906, 2792191, 16762993, 5766954, 16318226, 15517125, 13290186, 10197915, 7442943, 11316396, 9743236, 16757617, 16767648, 6618880, 16711680, 16860, 16860, 16773906, 65421, 2789375, 13714175, 12827549, 10595204, 7641720, 6062466, 8025242, 11507131, 10386594, 786176, 8584960, 16318208, 16731648, 16755616, 16734715, 14399157, 16754801, 16714752, 10026888, 3524608]
            n249 = Random Number (0-1)() -> (number: 0 to 1=w527:dbl)
            n250 = Random Number (0-1)() -> (number: 0 to 1=w519:dbl)
            n251 = Array Size(array=w516) -> (size(s)=w518:i32)
            n252 = Build Array (concatenate)(w516, u32[] [10427904, 10442496, 10444544, 10452224, 10458112, 5927680, 3633920, 1351424, 35084, 40813, 16959, 19615, 1376393, 4194441, 10748084, 10420349, 7536704, 8978459, 5963776, 3882593, 4944486, 5204291, 7553536, 5263440, 4013373, 2763306, 6447714, 9540204, 6982244, 5470832, 6056066, 40848, 11010228]) -> (w525:u32[])
            n253 = Array Size(array=w525) -> (size(s)=w528:i32)
            n254 = Multiply(x=w518, y=w519) -> (x*y=w520:dbl)
            n255 = Multiply(x=w528, y=w527) -> (x*y=w526:dbl)
            n256 = Round Toward -Infinity(1:w520) -> (0:w517:dbl)
            n257 = Round Toward -Infinity(1:w526) -> (0:w524:dbl)
            n258 = Index Array(array=w516, index=w517) -> (element=w510:u32)
            n259 = Index Array(array=w525, index=w524) -> (element=w512:u32)
            n260 = Greater?(x=w524, y=w518) -> (0:w523:bool)
            n261 = Select(t=u32 16777215, s=w523, f=u32 0) -> (s? t:f=w511:u32)
            n262 = Bundle By Name(cluster=w513, "Color"=u32 0) -> ()  [unwired: 1 out]
            n263 = Bundle By Name(cluster=w513, "Color"=w512) -> (w509:T3)
            n264 = Bundle By Name(cluster=w513, "Color"=w511) -> (w508:T3)
            n265 = Bundle By Name(cluster=w513, "Color"=w510) -> ()  [unwired: 1 out]
            n266 = local write "HeaderBk"(w509) -> ()
            n267 = local write "HeaderText"(w508) -> ()
          }
          frame "UpdateLastHeaders" {
            n268 = Unbundle By Name(w540) -> ("Header"=w531:u8[][], "Headers"=w537:cluster{"Header":u8[][]}[], "Names"=w536:string[])
            n269 = for {
              tunnel: w537 -> [w574] mode=indexing
              tunnel: w531 -> [w572]
              tunnel: [w571] -> w539
              tunnel: [w570] -> w538
              i -> [w570]
              stop <- w571 stop-if-true
              n270 = Unbundle By Name(w574) -> ("Header"=w573:u8[][])
              n271 = Equal?(x=w572, y=w573) -> (x = y?=w571:bool)
            }
            n272 = case shown="False" w539 {
              tunnel: w538 -> [_ w556]
              tunnel: w537 -> [w547 w555]
              tunnel: w536 -> [w545 w554]
              tunnel: w535 -> [w544 w553]
              tunnel: w534 -> [w543 w552]
              tunnel: w531 -> [w542 _]
              frame False {
                n273 = Bundle("Header"=w542) -> (w541:cluster{"Header":u8[][]})  [unwired: 1 in]
                n274 = local read "Text"() -> (w546:string)
                n275 = Build Array (concatenate)(w546, w545) -> (w551:string[])
                n276 = Build Array (concatenate)(w541, w547) -> (w550:cluster{"Header":u8[][]}[])
                n277 = Bundle By Name(cluster=w544, "Headers"=w550, "Names"=w551) -> (w549:T4)
                n278 = Flatten To String(anything=w549) -> (data string=w548:string)  [unwired: 3 in, 2 out]
                n279 = Write to Text File(file (use dialog)=w543, text=w548) -> ()  [unwired: 2 in, 3 out]
              }
              frame True {
                n280 = case shown="Default" w556 {
                  selector: w556 -> [_ w565]
                  tunnel: w555 -> [_ w569]
                  tunnel: w554 -> [_ w566]
                  tunnel: w553 -> [_ w562]
                  tunnel: w552 -> [_ w557]
                  frame 0 {
                  }
                  frame Default {
                    n281 = Delete From Array(array=w566, index=w565) -> (array with subset deleted=w564:string[])  [unwired: 1 in, 1 out]
                    n282 = Delete From Array(array=w569, index=w565) -> (deleted portion=w568:cluster{"Header":u8[][]}, array with subset deleted=w567:cluster{"Header":u8[][]}[])  [unwired: 1 in]
                    n283 = local read "Text"() -> (w563:string)
                    n284 = Build Array (concatenate)(w563, w564) -> (w561:string[])
                    n285 = Build Array (concatenate)(w568, w567) -> (w560:cluster{"Header":u8[][]}[])
                    n286 = Bundle By Name(cluster=w562, "Headers"=w560, "Names"=w561) -> (w559:T4)
                    n287 = Flatten To String(anything=w559) -> (data string=w558:string)  [unwired: 3 in, 2 out]
                    n288 = Write to Text File(file (use dialog)=w557, text=w558) -> ()  [unwired: 2 in, 3 out]
                  }
                }
              }
            }
          }
        }
        n289 = Equal?(x=w53, y="Exit") -> (x = y?=w56:bool)
        n290 = Select(t="Error", s=w52, f=w53) -> (s? t:f=w57:string)
      }
    }
    frame Error {
    }
  }
  "error out" <- w12
  n291 = stacked-sequence {
    tunnel: w12 -> [_]
    tunnel: [w578] -> w11
    tunnel: [w576] -> w10
    frame #0 {
      n292 = local read "Thickness (pixels)"() -> (w578:u8)
      n293 = local read "Frame"() -> (w577:T3)
      n294 = Unbundle By Name(w577) -> ("Color"=w576:u32)
    }
  }
  "FrameColorOut" <- w10
  "FrameThicknessOut" <- w11
  n295 = Unbundle By Name(w15) -> ("Cancel"=→"Cancelled":bool, "Header"=→"HeaderIconOut":u8[][])  [unwired: 1 out]
